vi "GlobalVariable.vi"() -> ()   [LabVIEW 2021]
uses:
  Global 1.vi
panel:
  out "Numeric 2":dbl
  out "Numeric":dbl
  out "Boolean":bool
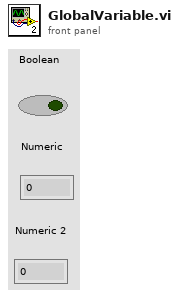
[diagram p1: front panel]
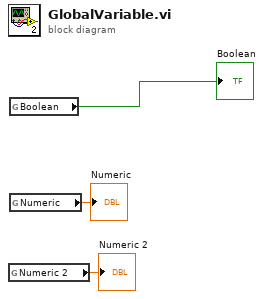
[diagram p0: block diagram]
diagram:
  n1 = global read "Global 1.vi" "Numeric 2"() -> (→"Numeric 2":dbl)
  n2 = global read "Global 1.vi" "Boolean"() -> (→"Boolean":bool)
  n3 = global read "Global 1.vi" "Numeric"() -> (→"Numeric":dbl)
